vi "HexU8_to_DecString.vi"(5 "String":string="0f 23", 7 "offset (0)":i32) -> (6 "decimal integer string":string)   [LabVIEW 2023]
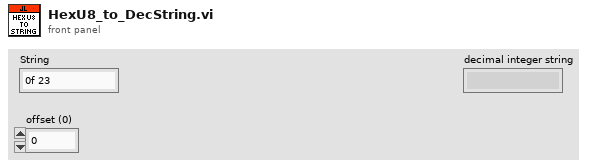
[diagram p1: front panel]
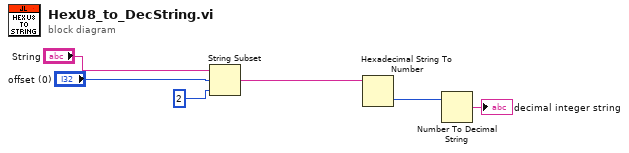
[diagram p0: block diagram]
diagram:
  n1 = String Subset(string="String", offset (0)="offset (0)", length (rest)=2 ("offset (0)")) -> (substring=w1:string)
  n2 = Hexadecimal String To Number(string=w1) -> (number=w4:u32)  [unwired: 2 in, 1 out]
  n3 = Number To Decimal String(number=w4) -> (decimal integer string=→"decimal integer string":string)  [unwired: 1 in]
